vi "viserver name.vi"() -> (3 "viserver vi name":string)   [LabVIEW 2013]
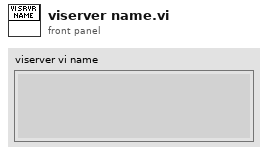
[diagram p1: front panel]
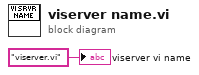
[diagram p0: block diagram]
diagram:
  "viserver vi name" <- "viserver.vi" ("name or relative path")
